vi "FreeCOM.vi"() -> ()   [LabVIEW 2012]
uses:
  <vilib>/Instr/_visa.llb/VISA Configure Serial Port (Serial Instr).vi
panel:
  out "Ram":string
  in  "保存数据":bool
  in  "清空接收区":bool
  in  "清空波形区":bool
  in  "清空计数":bool
  out "RX":dbl
  out "TX":dbl
  in  "换行":bool
  in  "send":bool
  in  "发送区":string
  out "串口波形图":dbl(graph)
  out "接收区":string
  in  "端口号":u16(ring) caption="Port" items=["COM1", "COM2", "COM3", "COM4", "COM5"]
  in  "波特率":u16(ring) caption="Baud" items=["9600", "115200"]
  out "串口状态":bool
  in  "exit":bool
  in  "open":bool
  # "Count"
  # "Config"
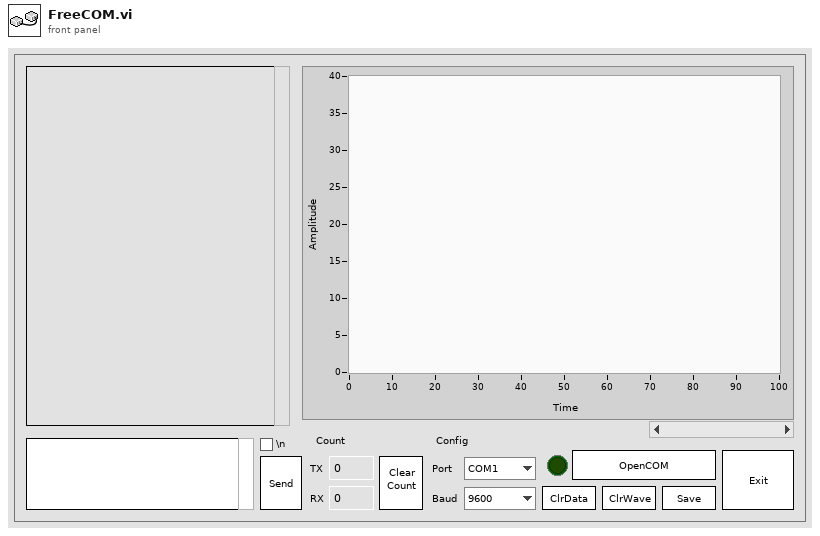
[diagram p1: front panel]
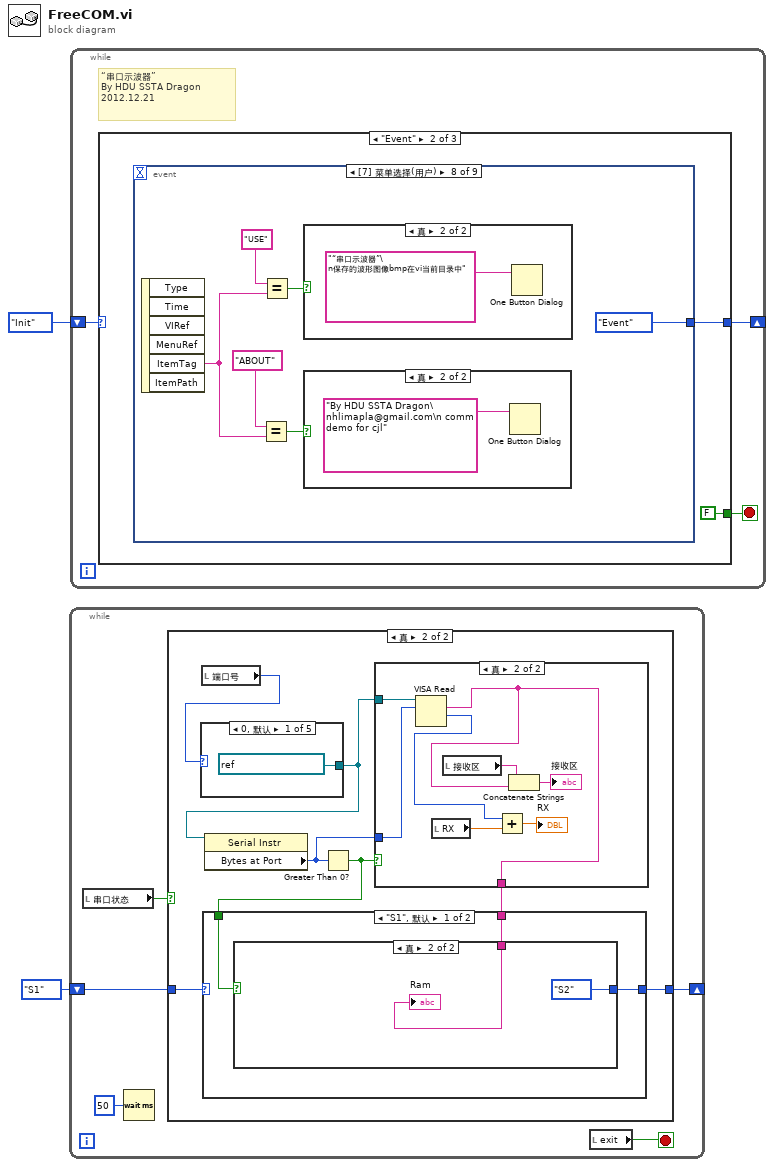
[diagram p0: block diagram]
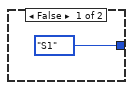
[diagram p2: hidden frame]
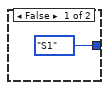
[diagram p3: hidden frame]
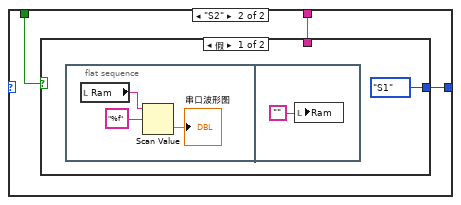
[diagram p4: hidden frame]
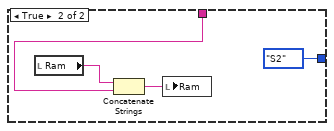
[diagram p5: hidden frame]
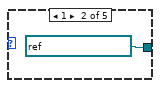
[diagram p7: hidden frame]
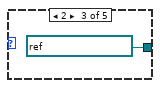
[diagram p8: hidden frame]
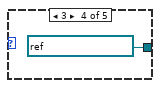
[diagram p9: hidden frame]
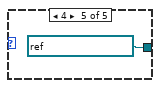
[diagram p10: hidden frame]
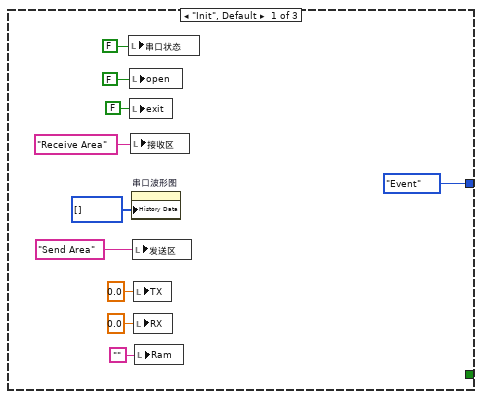
[diagram p11: hidden frame]
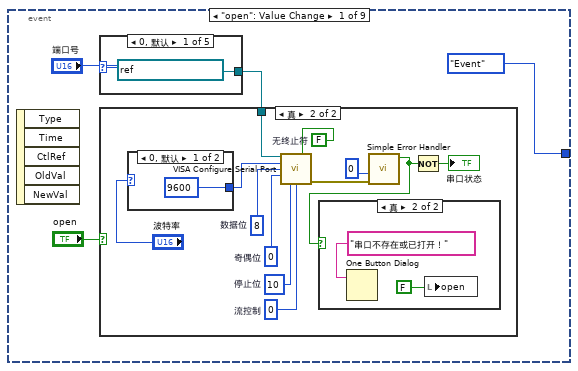
[diagram p12: hidden frame]
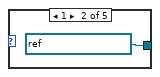
[diagram p13: hidden frame]
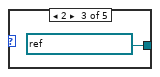
[diagram p14: hidden frame]
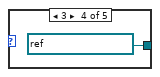
[diagram p15: hidden frame]
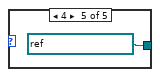
[diagram p16: hidden frame]
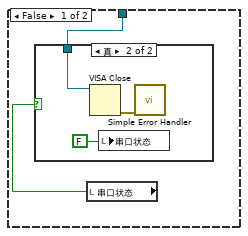
[diagram p17: hidden frame]
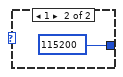
[diagram p20: hidden frame]
diagram:
  n1 = while {
    shift-right: [w3] -> _
    shift-left: enum16{"S1", "S2"}."S1" -> [w4]
    stop <- w6 stop-if-true
    n2 = local read "串口状态"() -> (w7:bool)
    n3 = Wait (ms)(milliseconds to wait=u32 50 ("等待时间（毫秒）")) -> ()  [unwired: 1 out]
    n4 = case shown="真" w7 {
      tunnel: w4 -> [_ w12]
      tunnel: [enum16{"S1", "S2"}."S1" w9] -> w3
      frame False {
      }
      frame True {
        n5 = local read "端口号"() -> (w15:u16)
        n6 = case shown="0, 默认" w15 {
          tunnel: [refnum<visa-resource-name> "ASRL1::INSTR" ("VISA resource name") refnum<visa-resource-name> "ASRL2::INSTR" ("VISA resource name") refnum<visa-resource-name> "ASRL3::INSTR" ("VISA resource name") refnum<visa-resource-name> "ASRL4::INSTR" ("VISA resource name") refnum<visa-resource-name> "ASRL5::INSTR" ("VISA resource name")] -> w14
          frame 0, Default {
          }
          frame 1 {
          }
          frame 2 {
          }
          frame 3 {
          }
          frame 4 {
          }
        }
        n7 = property class="Serial Instr"(reference=w14) -> ("Bytes at Port"=w13:u32)  [unwired: 1 in, 2 out]
        n8 = Greater Than 0?(x=w13) -> (x > 0?=w11:bool)
        n9 = case shown="真" w11 {
          tunnel: w14 -> [_ w41]
          tunnel: w13 -> [_ w36]
          tunnel: [_ w35] -> w10
          frame False {
          }
          frame True {
            n10 = VISA Read(VISA resource name=w41, byte count=w36) -> (read buffer=w35:string, return count=w34:u32)  [unwired: 1 in, 2 out]
            n11 = local read "RX"() -> (w38:dbl)
            n12 = local read "接收区"() -> (w39:string)
            n13 = Add(x=w34, y=w38) -> (x+y=→"RX":dbl)
            n14 = Concatenate Strings(w39, w35) -> (→"接收区":string)
          }
        }
        n15 = case shown="\"S1\", 默认" w12 {
          tunnel: w11 -> [w18 w24]
          tunnel: w10 -> [w17 w22]
          tunnel: [w16 w23] -> w9
          frame "S1", Default {
            n16 = case shown="真" w18 {
              tunnel: w17 -> [_ w21]
              tunnel: [enum16{"S1", "S2"}."S1" enum16{"S1", "S2"}."S2"] -> w16
              frame False {
              }
              frame True {
                "Ram" <- w21
              }
            }
          }
          frame "S2" {
            n17 = case shown="假" w24 {
              tunnel: [enum16{"S1", "S2"}."S1" enum16{"S1", "S2"}."S2"] -> w23
              tunnel: w22 -> [_ w30]
              frame False {
                n18 = flat-sequence {
                  frame #0 {
                    n19 = local read "Ram"() -> (w26:string)
                    n20 = Scan Value(string=w26, format string="%f" ("格式字符串")) -> (value=→"串口波形图":dbl)  [unwired: 1 in, 1 out]
                  }
                  frame #1 {
                    n21 = local write "Ram"("") -> ()
                  }
                }
              }
              frame True {
                n22 = local read "Ram"() -> (w31:string)
                n23 = Concatenate Strings(w31, w30) -> (w32:string)
                n24 = local write "Ram"(w32) -> ()
              }
            }
          }
        }
      }
    }
    n25 = local read "exit"() -> (w6:bool)
  }
  n26 = while {
    shift-right: [w47] -> _
    shift-left: enum16{"Init", "Event", "Exit"}."Init" -> [w48]
    stop <- w49 stop-if-true
    # "“串口示波器”\nBy HDU SSTA Dragon\n2012.12.21"
    n27 = case shown="\"Event\"" w48 {
      tunnel: [_ FALSE TRUE] -> w49
      tunnel: [enum16{"Init", "Event", "Exit"}."Event" w60 enum16{"Init", "Event", "Exit"}."Exit"] -> w47
      frame "Init", Default {
        n28 = local write "串口状态"(FALSE) -> ()
        n29 = local write "open"(FALSE) -> ()
        n30 = local write "exit"(FALSE ("exit")) -> ()
        n31 = local write "接收区"("Receive Area") -> ()
        n32 = property on="串口波形图" class="WFChart (严格)"("History Data"=u8[] [] ("历史数据")) -> ()  [unwired: 2 in, 2 out]
        n33 = local write "发送区"("Send Area" ("发送区")) -> ()
        n34 = local write "TX"(0.0 ("TX")) -> ()
        n35 = local write "RX"(0.0 ("RX")) -> ()
        n36 = local write "Ram"("") -> ()
      }
      frame "Event" {
        n37 = event shown="[7] 菜单选择(用户)" {
          selector: _ -> [_ _ _ _ _ _ _ _ _]
          dyn-events: _ -> [_ _ _ _ _ _ _ _ _]
          timeout: _ -> [_ _ _ _ _ _ _ _ _]
          tunnel: [enum16{"Init", "Event", "Exit"}."Event" enum16{"Init", "Event", "Exit"}."Event" enum16{"Init", "Event", "Exit"}."Event" enum16{"Init", "Event", "Exit"}."Event" enum16{"Init", "Event", "Exit"}."Event" enum16{"Init", "Event", "Exit"}."Event" enum16{"Init", "Event", "Exit"}."Event" enum16{"Init", "Event", "Exit"}."Event" enum16{"Init", "Event", "Exit"}."Exit"] -> w60
          event "open": Value Change {
            n38 = event-data() -> ()  [unwired: 1 in, 5 out]
            n39 = case shown="0, 默认" "端口号" {
              tunnel: [refnum<visa-resource-name> "ASRL1::INSTR" ("VISA resource name") refnum<visa-resource-name> "ASRL2::INSTR" ("VISA resource name") refnum<visa-resource-name> "ASRL3::INSTR" ("VISA resource name") refnum<visa-resource-name> "ASRL4::INSTR" ("VISA resource name") refnum<visa-resource-name> "ASRL5::INSTR" ("VISA resource name")] -> w64
              frame 0, Default {
              }
              frame 1 {
              }
              frame 2 {
              }
              frame 3 {
              }
              frame 4 {
              }
            }
            n40 = case shown="真" "open" {
              tunnel: w64 -> [w72 w77]
              frame False {
                n41 = local read "串口状态"() -> (w71:bool)
                n42 = case shown="真" w71 {
                  tunnel: w72 -> [_ w73]
                  frame False {
                  }
                  frame True {
                    n43 = VISA Close(VISA resource name=w73) -> (error out=w75:errorcluster)  [unwired: 1 in]
                    n44 = local write "串口状态"(FALSE) -> ()
                    n45 = call <vilib>:"Simple Error Handler.vi"("error in (no error)"=w75) -> ()  [unwired: 4 in, 5 out]
                  }
                }
              }
              frame True {
                w78 = FALSE  # 无终止符
                w85 = u16 0  # 流控制
                w84 = u16 10  # 停止位
                w83 = u8 0  # 奇偶位
                w82 = u16 8  # 数据位
                n46 = case shown="0, 默认" "波特率" {
                  tunnel: [u32 9600 u32 115200] -> w81
                  frame 0, Default {
                  }
                  frame 1 {
                  }
                }
                n47 = call-poly "VISA Configure Serial Port"("VISA resource name"=w77, "Enable Termination\nChar (T)"=w78, "baud rate (9600)"=w81, "data bits (8)"=w82, "parity (0:none)"=w83, "stop bits (10: 1 bit)"=w84, "flow control (0:none)"=w85) -> ("error out"=w86:errorcluster)  [unwired: 7 in, 1 out]
                n48 = call <vilib>:"Simple Error Handler.vi"("type of dialog (OK msg:1)"=0, "error in (no error)"=w86) -> ("error?"=w79:bool)  [unwired: 3 in, 4 out]
                n49 = case shown="真" w79 {
                  frame False {
                  }
                  frame True {
                    n50 = One Button Dialog(message="串口不存在或已打开！") -> ()  [unwired: 1 in, 1 out]
                    n51 = local write "open"(FALSE) -> ()
                  }
                }
                n52 = Not(x=w79) -> (.not. x?=→"串口状态":bool)
              }
            }
          }
          event "端口号", "波特率": Value Change {
            n53 = event-data() -> ("OldVal"=w93:u16)  [unwired: 1 in, 4 out]
            n54 = local read "串口状态"() -> (w94:bool)
            n55 = case shown="真" w94 {
              tunnel: w93 -> [_ w95]
              frame False {
              }
              frame True {
                n56 = flat-sequence {
                  tunnel: w95 -> [w100]
                  frame #0 {
                    n57 = case shown="0, 默认" w100 {
                      tunnel: [refnum<visa-resource-name> "ASRL1::INSTR" ("VISA resource name") refnum<visa-resource-name> "ASRL2::INSTR" ("VISA resource name") refnum<visa-resource-name> "ASRL3::INSTR" ("VISA resource name") refnum<visa-resource-name> "ASRL4::INSTR" ("VISA resource name") refnum<visa-resource-name> "ASRL5::INSTR" ("VISA resource name")] -> w97
                      frame 0, Default {
                      }
                      frame 1 {
                      }
                      frame 2 {
                      }
                      frame 3 {
                      }
                      frame 4 {
                      }
                    }
                    n58 = VISA Close(VISA resource name=w97) -> (error out=w99:errorcluster)  [unwired: 1 in]
                    n59 = call <vilib>:"Simple Error Handler.vi"("error in (no error)"=w99) -> ()  [unwired: 4 in, 5 out]
                    n60 = local write "串口状态"(FALSE) -> ()
                    n61 = local write "open"(FALSE ("open")) -> ()
                  }
                }
              }
            }
          }
          event "send": Mouse Down {
            n62 = event-data() -> ()  [unwired: 1 in, 7 out]
            n63 = local read "串口状态"() -> (w107:bool)
            n64 = case shown="真" w107 {
              frame False {
              }
              frame True {
                n65 = local read "端口号"() -> (w117:u16)
                n66 = case shown="真" "换行" {
                  tunnel: [_ "\r"] -> w115
                  tunnel: [_ "\n"] -> w114
                  frame False {
                  }
                  frame True {
                  }
                }
                n67 = case shown="0, 默认" w117 {
                  tunnel: [refnum<visa-resource-name> "ASRL1::INSTR" ("VISA resource name") refnum<visa-resource-name> "ASRL2::INSTR" ("VISA resource name") refnum<visa-resource-name> "ASRL3::INSTR" ("VISA resource name") refnum<visa-resource-name> "ASRL4::INSTR" ("VISA resource name") refnum<visa-resource-name> "ASRL5::INSTR" ("VISA resource name")] -> w116
                  frame 0, Default {
                  }
                  frame 1 {
                  }
                  frame 2 {
                  }
                  frame 3 {
                  }
                  frame 4 {
                  }
                }
                n68 = Concatenate Strings("发送区", w115, w114) -> (w111:string)
                n69 = local read "TX"() -> (w110:dbl)
                n70 = VISA Write(VISA resource name=w116, write buffer=w111) -> (return count=w108:u32)  [unwired: 1 in, 2 out]
                n71 = Add(x=w108, y=w110) -> (x+y=→"TX":dbl)
              }
            }
          }
          event "清空计数": Mouse Down {
            n72 = event-data() -> ()  [unwired: 1 in, 7 out]
            n73 = local write "RX"(0.0 ("RX")) -> ()
            n74 = local write "TX"(0.0 ("TX")) -> ()
          }
          event "清空接收区": Mouse Down {
            n75 = event-data() -> ()  [unwired: 1 in, 7 out]
            n76 = local write "接收区"("") -> ()
          }
          event "清空波形区": Mouse Down {
            n77 = event-data() -> ()  [unwired: 1 in, 7 out]
            n78 = property on="串口波形图" class="WFChart (严格)"("History Data"=u8[] [] ("历史数据")) -> ()  [unwired: 2 in, 2 out]
          }
          event "保存数据": Mouse Down {
            n79 = event-data() -> ()  [unwired: 1 in, 7 out]
            n80 = Current VI's Path() -> (path=w132:path)
            n81 = invoke on="串口波形图" class="WFChart (严格)" method="Export Image"("FileType"=enum32{"BMP", "EPS", "EMF", "PICT"}."BMP" ("文件类型"), "Target"=enum32{"File", "Clipboard"}."File" ("目标"), "Path"=w132) -> ()  [unwired: 5 in, 8 out]
          }
          event Menu Selection (User) {
            n82 = event-data() -> ("ItemTag"=w139:string)  [unwired: 1 in, 5 out]
            n83 = Equal?(x="ABOUT", y=w139) -> (x = y?=w140:bool)
            n84 = Equal?(x="USE", y=w139) -> (x = y?=w141:bool)
            n85 = case shown="真" w141 {
              frame False {
              }
              frame True {
                n86 = One Button Dialog(message="“串口示波器”\n保存的波形图像bmp在vi当前目录中" ("Message")) -> ()  [unwired: 1 in, 1 out]
              }
            }
            n87 = case shown="真" w140 {
              frame False {
              }
              frame True {
                n88 = One Button Dialog(message="By HDU SSTA Dragon\nhlimapla@gmail.com\n comm demo for cjl" ("Message")) -> ()  [unwired: 1 in, 1 out]
              }
            }
          }
          event "exit": Value Change {
            n89 = event-data() -> ()  [unwired: 1 in, 5 out]
            n90 = local read "串口状态"() -> (w147:bool)
            n91 = local read "端口号"() -> (w145:u16)
            n92 = case shown="0, 默认" w145 {
              tunnel: [refnum<visa-resource-name> "ASRL1::INSTR" ("VISA resource name") refnum<visa-resource-name> "ASRL2::INSTR" ("VISA resource name") refnum<visa-resource-name> "ASRL3::INSTR" ("VISA resource name") refnum<visa-resource-name> "ASRL4::INSTR" ("VISA resource name") refnum<visa-resource-name> "ASRL5::INSTR" ("VISA resource name")] -> w146
              frame 0, Default {
              }
              frame 1 {
              }
              frame 2 {
              }
              frame 3 {
              }
              frame 4 {
              }
            }
            n93 = case shown="真" w147 {
              tunnel: w146 -> [_ w156]
              frame False {
              }
              frame True {
                n94 = VISA Close(VISA resource name=w156) -> (error out=w155:errorcluster)  [unwired: 1 in]
                n95 = local write "串口状态"(FALSE) -> ()
                n96 = local write "open"(FALSE) -> ()
                n97 = call <vilib>:"Simple Error Handler.vi"("error in (no error)"=w155) -> ()  [unwired: 4 in, 5 out]
              }
            }
          }
        }
      }
      frame "Exit" {
      }
    }
  }
